vi "Plane Coordinate Generator.vi"(8 "error in (no error)":errorcluster, 10 "AcquireZplane Index":i32, 11 "AOL_Globals":T1={"Imaging Protocol"=enum."AOL Z-Stack", "Number of POI"=0, "Number of Miniscans"=0, "Number of Trials"=0, "Number of Cycles "=0, "# Averaged Frames"=0, "Laser power (%)"=0, "Pockels"=0.0, "Acquisition Length (sec)"=0.0, "Fill time (us)"=0.0, "POI Dwell time (us)"=0.0, "Miniscan Dwell time per pixel (us)"=0.0, "PMT 1"=0.0, "PMT 2"=0.0, "Back Apperture"=512.0, "Frame Size"=0, "Center Frequency"=0.0, "Field of View"=0.0, "DwellTime (us)"=0.0, "Wavelength (nm)"=0.0, "Zoom"=0.0, "AOL Z"=0.0, "AOL Mode"=enum."Raster", "GridXY"=0.0, "GridZ"=0.0, "TriggerPeriod (sec)"=0.0, "Number of Pixels in Miniscan"=0, "Experiment folder path"=path "", "X centre"=0.0, "Y centre"=0.0, "Angle (degrees)"=0.0, "Plane Mode"=0, "Threshold"=[], "Regenerate Chirps"=FALSE, "Rectangle ROI length (pixels)"=0, "Rectangle ROI height (pixels)"=0, "AOD fill"=0, "Samples Wait after Trigger"=0, "StartUp Delay"=0, "Slip Cycle"=163840, "Add Cycle"=FALSE} {"Plane Mode" items=["XY Plane"]; "Frame Size" items=["100X100"=100, "128X128"=128, "200X200"=200, "256X256"=256, "512X512"=512, "1024x1024"=1024, "2048x2048"=2048]; "Back Apperture" format="%#.6g"; "Pockels" format="%#.6g"; "PMT 2" format="%#.6g"; "PMT 1" format="%#.6g"; "Angle (degrees)" format="%#.6g"; "POI Dwell time (us)" format="%#.6g"}) -> (0 "error out":errorcluster, 3 "ROI Attributes (broken down to miniscans)":T6)   [LabVIEW 2013]
uses:
  Typedefs/ROI XY coordinates cluster.ctl
  Typedefs/Controls/AOL_Globals.ctl
  Typedefs/Imaging Protocols enum.ctl
  Typedefs/Frame Size.ctl
  Typedefs/AOL modes.ctl
  Typedefs/Plane Mode.ctl
  User Interface/Visualisation/Functional Imaging Viewer/Typedefs/ROI parameters data type.ctl
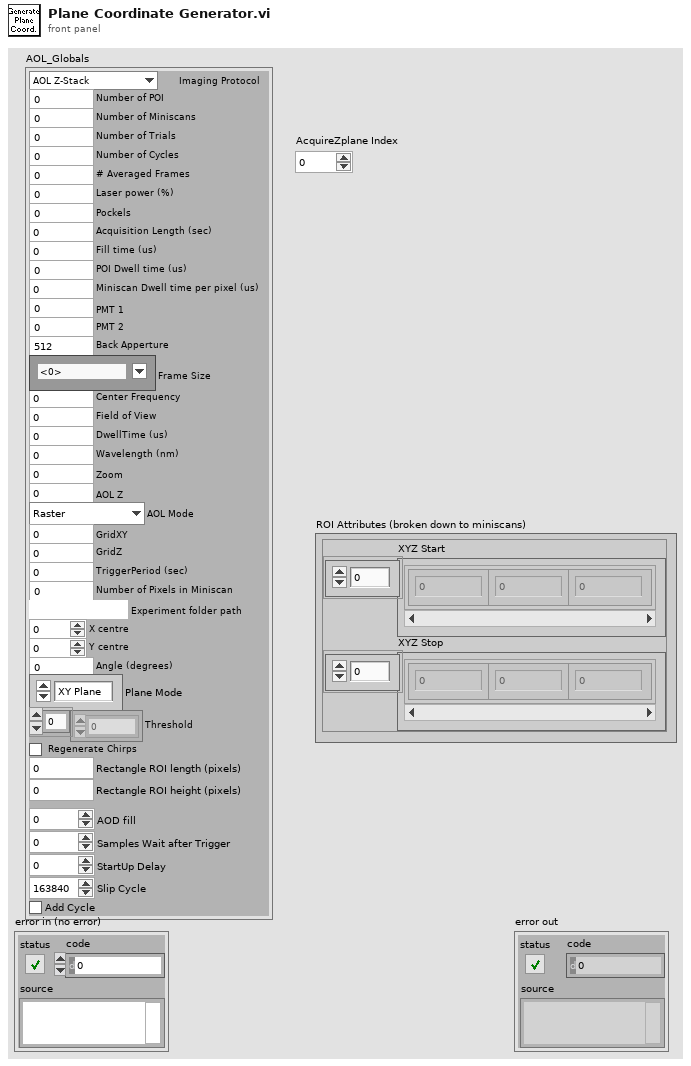
[diagram p1: front panel]
types:
  T1 = typedef "AOL_Globals.ctl" = cluster{"Imaging Protocol":T2, "Number of POI":u16, "Number of Miniscans":u16, "Number of Trials":u16, "Number of Cycles ":u64, "# Averaged Frames":u16, "Laser power (%)":u8, "Pockels":dbl, "Acquisition Length (sec)":dbl, "Fill time (us)":dbl, "POI Dwell time (us)":dbl, "Miniscan Dwell time per pixel (us)":dbl, "PMT 1":dbl, "PMT 2":dbl, "Back Apperture":dbl, "Frame Size":T3, "Center Frequency":dbl, "Field of View":dbl, "DwellTime (us)":dbl, "Wavelength (nm)":dbl, "Zoom":dbl, "AOL Z":dbl, "AOL Mode":T4, "GridXY":dbl, "GridZ":dbl, "TriggerPeriod (sec)":dbl, "Number of Pixels in Miniscan":u16, "Experiment folder path":path, "X centre":dbl, "Y centre":dbl, "Angle (degrees)":dbl, "Plane Mode":T5, "Threshold":u16[], "Regenerate Chirps":bool, "Rectangle ROI length (pixels)":u16, "Rectangle ROI height (pixels)":u16, "AOD fill":u16, "Samples Wait after Trigger":u16, "StartUp Delay":i32, "Slip Cycle":u32, "Add Cycle":bool}
  T2 = typedef "Imaging Protocols enum.ctl" = enum16{"AOL Z-Stack", "Motor Z Stack", "Functional Acquisition", "Single Plane Acquisition", "Volume Acquisition", "Live Imaging", "Live Plane Imaging", "Live Volume Imaging"}
  T3 = typedef "Frame Size.ctl" = u16
  T4 = typedef "AOL modes.ctl" = enum16{"Raster", "Structural", "Pointing", "Mini Scan", "Alignment"}
  T5 = typedef "Plane Mode.ctl" = u16
  T6 = typedef "ROI XY coordinates cluster.ctl" = cluster{"XYZ Start":cluster{"X":sgl, "Y":sgl, "Z":sgl}[], "XYZ Stop":cluster{"X":sgl, "Y":sgl, "Z":sgl}[]}
  T7 = typedef "ROI parameters data type.ctl" = cluster{"ROI index":dbl, "ROI ID":dbl, "ROI Time (ns)":dbl, "Pixels in ROI":dbl, "X start":dbl, "Y start":dbl, "Z start":dbl, "X stop":dbl, "Y stop":dbl, "Z stop":dbl, "Angle (deg)":dbl, "Composite ID":dbl, "Number of lines":dbl, "Frame Size":dbl, "Zoom":dbl, "Laser Power (%)":dbl, "ROI group ID":dbl}
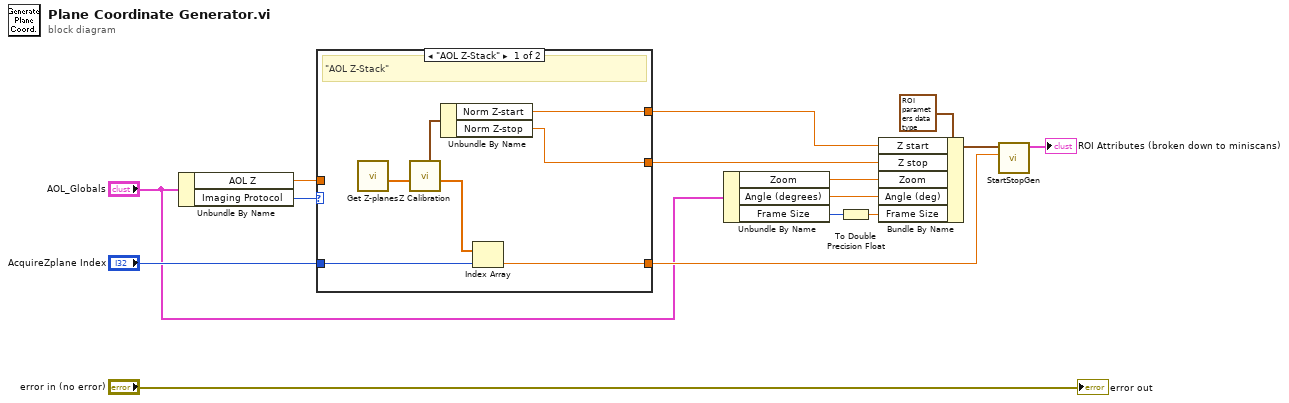
[diagram p0: block diagram]
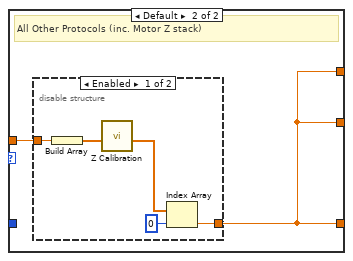
[diagram p2: hidden frame]
diagram:
  n1 = Unbundle By Name("AOL_Globals") -> ("AOL Z"=w7:dbl, "Imaging Protocol"=w8:T2)
  n2 = case shown="\"AOL Z-Stack\"" w8 {
    tunnel: [w16 w24] -> w14
    tunnel: [w17 w24] -> w13
    tunnel: "AcquireZplane Index" -> [w22 _]
    tunnel: [w21 w24] -> w10
    tunnel: w7 -> [_ w23]
    frame "AOL Z-Stack" {
      # "\"AOL Z-Stack\""
      n3 = call "Get Z-planes.vi"() -> ("Z Planes(um)"=w20:dbl[])  [unwired: 7 in, 4 out]
      n4 = call "Z Calibration.vi"("Z Planes"=w20) -> ("Norm Z"=w19:dbl[], "Norm Z start/stop"=w18:cluster{"Norm Z-start":dbl, "Norm Z-stop":dbl})  [unwired: 7 in, 2 out]
      n5 = Unbundle By Name(w18) -> ("Norm Z-start"=w17:dbl, "Norm Z-stop"=w16:dbl)
      n6 = Index Array(array=w19, index=w22) -> (element=w21:dbl)
    }
    frame Default {
      # "All Other Protocols (inc. Motor Z stack)"
      n7 = disable-structure shown="Enabled" {
        disable-tunnel: [w26 w30] -> w24
        disable-tunnel: w23 -> [w25 w30]
        frame Enabled {
          n8 = Build Array(w25) -> (w29:dbl[])
          n9 = call "Z Calibration.vi"("Z Planes"=w29) -> ("Norm Z"=w28:dbl[])  [unwired: 7 in, 3 out]
          n10 = Index Array(array=w28, index=0) -> (element=w26:dbl)
        }
        frame Disabled {
        }
      }
    }
  }
  n11 = Unbundle By Name("AOL_Globals") -> ("Zoom"=w3:dbl, "Angle (degrees)"=w2:dbl, "Frame Size"=w1:T3)
  n12 = To Double Precision Float(number=w1) -> (double precision float=w4:dbl)
  n13 = Bundle By Name(cluster=T7 {"ROI index"=0.0, "ROI ID"=0.0, "ROI Time (ns)"=0.0, "Pixels in ROI"=0.0, "X start"=0.0, "Y start"=0.0, "Z start"=0.0, "X stop"=0.0, "Y stop"=0.0, "Z stop"=0.0, "Angle (deg)"=0.0, "Composite ID"=0.0, "Number of lines"=0.0, "Frame Size"=0.0, "Zoom"=0.0, "Laser Power (%)"=0.0, "ROI group ID"=0.0} ("X-Y-Z coordinates"), "Z start"=w13, "Z stop"=w14, "Zoom"=w3, "Angle (deg)"=w2, "Frame Size"=w4) -> (w12:T7)
  n14 = call "StartStopGen.vi"("AOLZ"=w10, "X-Y-Z coordinates"=w12) -> ("ROI Coordinates (broken down to miniscans)"=→"ROI Attributes (broken down to miniscans)":T6)  [unwired: 9 in]
  "error out" <- "error in (no error)"
